vi "Condition Terminal Attributes.vi"(8 "error in":errorcluster, 9 "VI":refnum<vi>, 10 "Terminals":T1) -> (0 "error out":errorcluster, 2 "Terminal Attributes":T2)   [LabVIEW 2025, in "_Rescript.lvlib"]
uses:
  _Rescript.lvlib
  Terminal Attributes.ctl
  Attributes.ctl
  Terminals.ctl
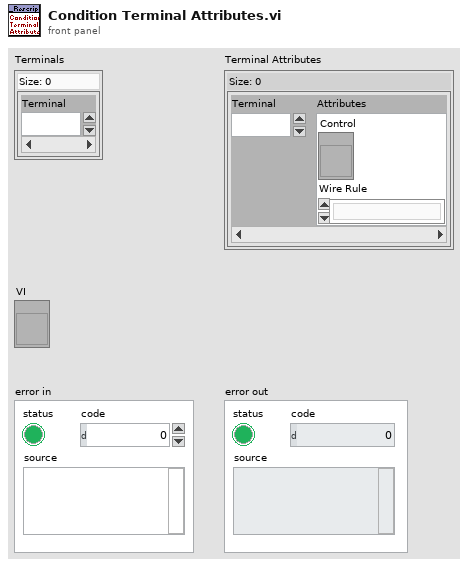
[diagram p1: front panel]
types:
  T1 = typedef "_Rescript.lvlib/Terminals.ctl" = set{i32}
  T2 = typedef "_Rescript.lvlib/Terminal Attributes.ctl" = map{i32, T3}
  T3 = typedef "_Rescript.lvlib/Attributes.ctl" = cluster{"Control":refnum<vi>, "Wire Rule":enum16{"Invalid Wire Rule", "Required", "Recommended", "Optional", "Dynamic Dispatch"}}
  T4 = enum16{"Invalid Wire Rule", "Required", "Recommended", "Optional", "Dynamic Dispatch"}[]
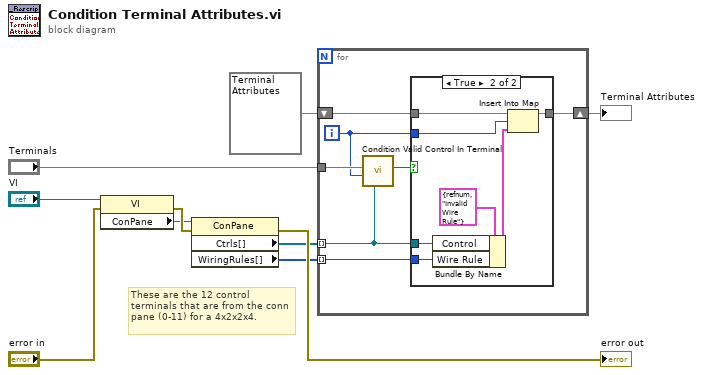
[diagram p0: block diagram]
diagram:
  # "These are the 12 control terminals that are from the conn pane (0-11) for a 4x2x2x4."
  n1 = property class="VI"(reference="VI", error in="error in") -> (error out=w9:errorcluster, "ConPane"=w8:refnum<vi>)  [unwired: 1 out]
  n2 = property class="ConPane"(reference=w8, error in=w9) -> (error out=→"error out":errorcluster, "Ctrls[]"=w4:refnum<vi>[], "WiringRules[]"=w3:T4)  [unwired: 1 out]
  n3 = for {
    tunnel: "Terminals" -> [w15]
    tunnel: w4 -> [w13] mode=indexing
    tunnel: w3 -> [w17] mode=indexing
    shift-right: [w12] -> w2
    shift-left: T2 {} ("Terminal Attributes") -> [w11]
    i -> [w14]
    n4 = call "Condition Valid Control In Terminal.vi"("Control"=w13, "Terminal"=w14, "Terminals"=w15) -> ("Valid"=w16:bool)  [unwired: 8 in]
    n5 = case shown="True" w16 {
      tunnel: w17 -> [_ w25]
      tunnel: w14 -> [_ w19]
      tunnel: w13 -> [_ w24]
      tunnel: [w18 w20] -> w12
      tunnel: w11 -> [w18 w21]
      frame False {
      }
      frame True {
        n6 = Bundle By Name(cluster=T3 {"Control"=refnum, "Wire Rule"=enum."Invalid Wire Rule"} ("value"), "Control"=w24, "Wire Rule"=w25) -> (w22:T3)
        n7 = Insert Into Map(map in=w21, key=w19, value=w22) -> (map out=w20:T2)  [unwired: 2 out]
      }
    }
  }
  "Terminal Attributes" <- w2
